vi "test_calibration.vi"() -> ()   [LabVIEW 2023]
panel:
  out "extended_video_device_list":string
  out "extended_audio_device_list":string
  out "calibration_pv":T1
  out "calibration_rm_depth_longthrow":T2
  out "calibration_rm_depth_ahat":T3
  out "calibration_rm_imu":cluster{"extrinsics":sgl[][]}
  out "calibration_rm_vlc":T4
  in  "framerate":u8=30
  in  "height":u16=1080
  in  "width":u16=1920
  in  "rm_imu_port":u16=3806
  in  "rm_vlc_port":u16=3800
  in  "host":string="192.168.1.7"
  in  "path in":path=path "C:/Users/jcds/Documents/GitHub/hl2ss/extensions/client_labview/hl2ss_labview/hl2ss_ulm.dll"
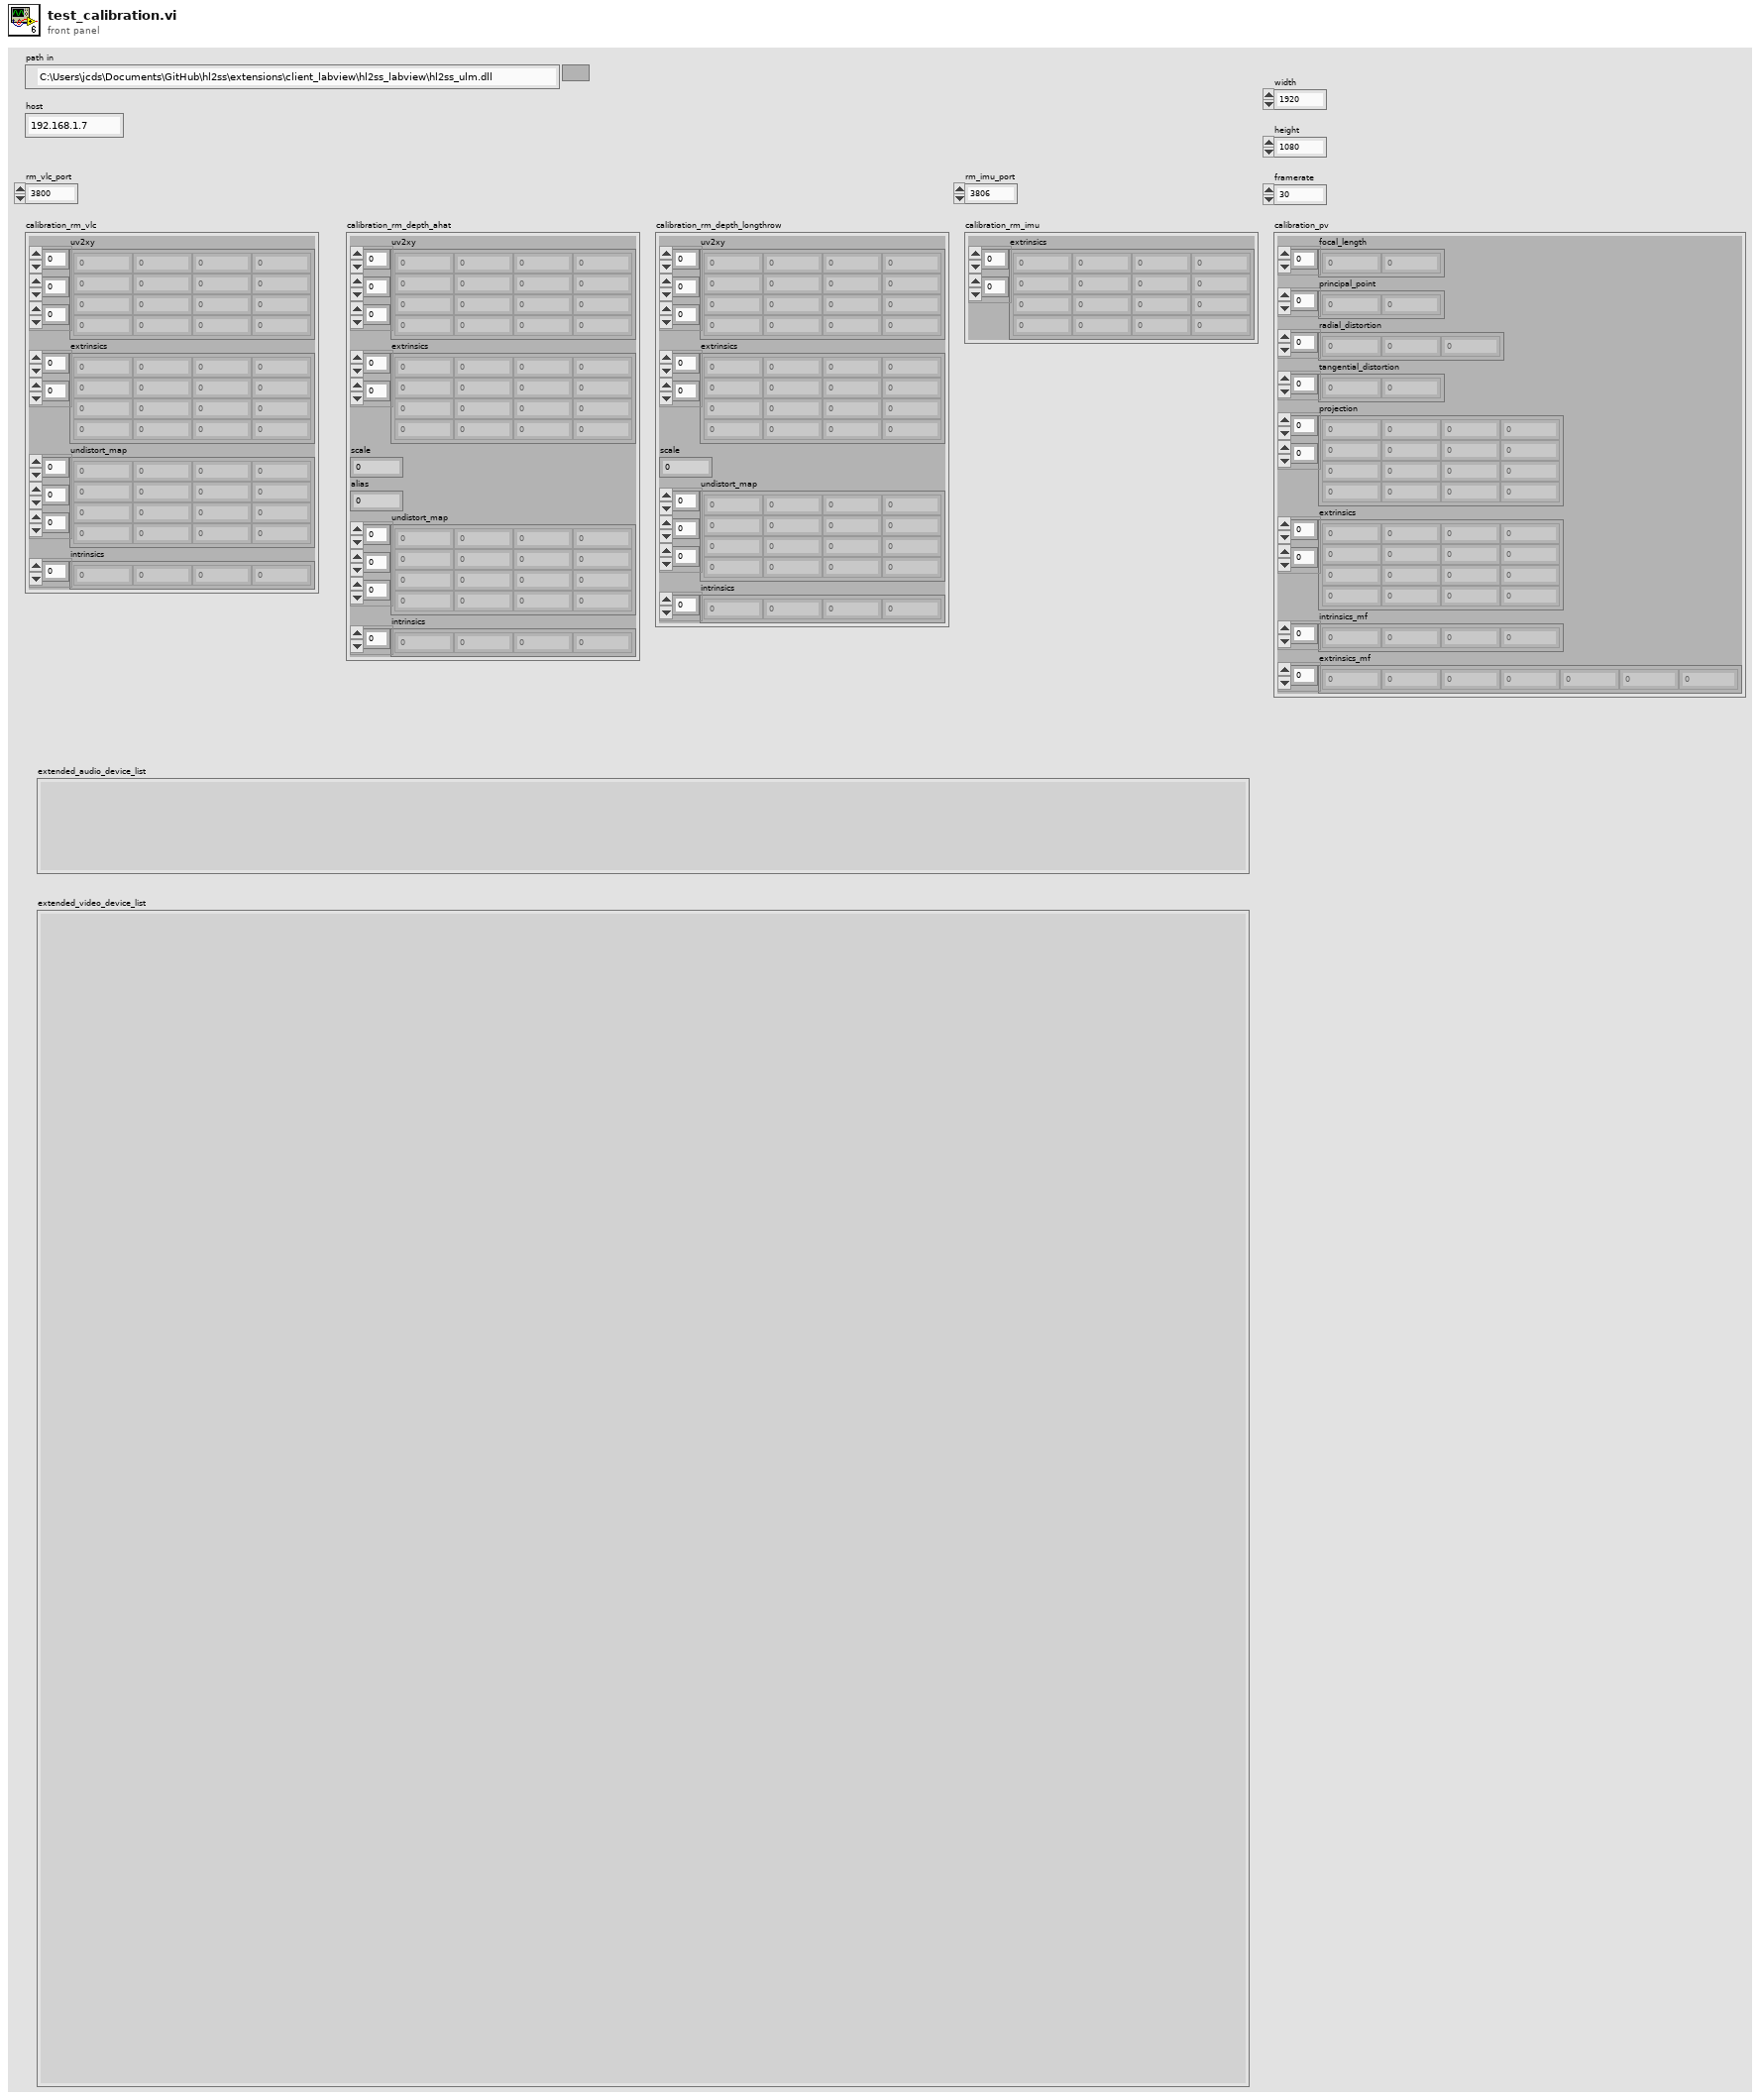
[diagram p1: front panel]
types:
  T1 = cluster{"focal_length":sgl[], "principal_point":sgl[], "radial_distortion":sgl[], "tangential_distortion":sgl[], "projection":sgl[][], "extrinsics":sgl[][], "intrinsics_mf":sgl[], "extrinsics_mf":sgl[]}
  T2 = cluster{"uv2xy":sgl[][][], "extrinsics":sgl[][], "scale":sgl, "undistort_map":sgl[][][], "intrinsics":sgl[]}
  T3 = cluster{"uv2xy":sgl[][][], "extrinsics":sgl[][], "scale":sgl, "alias":sgl, "undistort_map":sgl[][][], "intrinsics":sgl[]}
  T4 = cluster{"uv2xy":sgl[][][], "extrinsics":sgl[][], "undistort_map":sgl[][][], "intrinsics":sgl[]}
  T5 = cluster{"chunk":u64, "mixer_mode":u32, "loopback_gain":sgl, "microphone_gain":sgl, "profile":u8, "level":u8, "_reserved_0":u8, "_reserved_1":u8}
  T6 = cluster{"enable_mrc":u8, "hologram_composition":u8, "recording_indicator":u8, "video_stabilization":u8, "blank_protected":u8, "show_mesh":u8, "shared":u8, "_reserved_0":u8, "global_opacity":sgl, "output_width":sgl, "output_height":sgl, "video_stabilization_length":u32, "hologram_perspective":u32, "_reserved_1":u32}
  T7 = cluster{"chunk":u64, "mode":u8, "_reserved_0":u8, "width":u16, "height":u16, "framerate":u8, "divisor":u8, "profile":u8, "level":u8, "_reserved_1":u16, "bitrate":u32, "options_size":i64, "options_data":u64, "_reserved_2":u64}
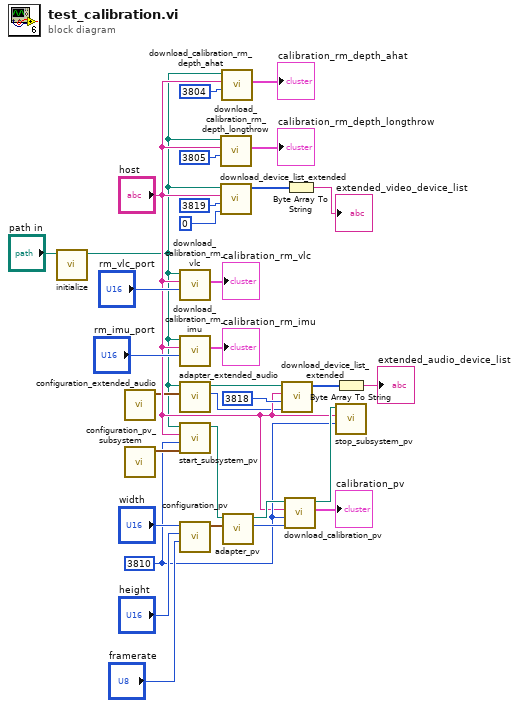
[diagram p0: block diagram]
diagram:
  w13 = u16 3810 ("port")
  n1 = call "initialize.vi"("path in"="path in") -> ("path out"=w1:path)  [unwired: 9 in, 1 out]
  n2 = call "configuration_extended_audio.vi"() -> ("configuration_extended_audio"=w2:T5)  [unwired: 11 in]
  n3 = call "configuration_pv_subsystem.vi"() -> ("configuration_pv_subsystem"=w31:T6)  [unwired: 11 in]
  n4 = call "download_calibration_rm_vlc.vi"("port"="rm_vlc_port", "host"="host", "path in"=w1) -> ("calibration"=→"calibration_rm_vlc":T4)  [unwired: 6 in, 2 out]
  n5 = call "download_calibration_rm_imu.vi"("port"="rm_imu_port", "host"="host", "path in"=w1) -> ("calibration"=→"calibration_rm_imu":cluster{"extrinsics":sgl[][]})  [unwired: 6 in, 2 out]
  n6 = call "adapter_extended_audio.vi"("configuration_extended_audio"=w2, "path in"=w1) -> ("configuration"=w4:u64, "path out"=w3:path)  [unwired: 8 in]
  n7 = call "start_subsystem_pv.vi"("configuration"=w31, "port"=w13, "host"="host", "path in"=w1) -> ("path out"=w29:path)  [unwired: 6 in, 1 out]
  n8 = call "configuration_pv.vi"("framerate"="framerate", "height"="height", "width"="width") -> ("configuration_pv"=w30:T7)  [unwired: 8 in]
  n9 = call "download_calibration_rm_depth_longthrow.vi"("port"=u16 3805, "host"="host", "path in"=w1) -> ("calibration"=→"calibration_rm_depth_longthrow":T2)  [unwired: 6 in, 2 out]
  n10 = call "download_device_list_extended.vi"("configuration"=u64 0, "port"=u16 3819, "host"="host", "path in"=w1) -> ("utf16_string"=w7:u8[])  [unwired: 6 in, 1 out]
  n11 = call "download_calibration_rm_depth_ahat.vi"("port"=u16 3804, "host"="host", "path in"=w1) -> ("calibration"=→"calibration_rm_depth_ahat":T3)  [unwired: 6 in, 2 out]
  n12 = call "adapter_pv.vi"("configuration_pv"=w30, "path in"=w29) -> ("configuration"=w20:u64, "path out"=w21:path)  [unwired: 8 in]
  n13 = call "download_device_list_extended.vi"("configuration"=w4, "port"=u16 3818, "host"="host", "path in"=w3) -> ("utf16_string"=w11:u8[])  [unwired: 6 in, 1 out]
  n14 = call "download_calibration_pv.vi"("configuration"=w20, "port"=w13, "host"="host", "path in"=w21) -> ("calibration"=→"calibration_pv":T1, "path out"=w14:path)  [unwired: 5 in, 1 out]
  n15 = Byte Array To String(unsigned byte array=w7) -> (string=→"extended_video_device_list":string)
  n16 = Byte Array To String(unsigned byte array=w11) -> (string=→"extended_audio_device_list":string)
  n17 = call "stop_subsystem_pv.vi"("port"=w13, "host"="host", "path in"=w14) -> ()  [unwired: 7 in, 2 out]
